vi "Construção string (salvar).vi"(8 "error in (no error)":errorcluster) -> (0 "error out":errorcluster, 2 "String":string)   [LabVIEW 2020]
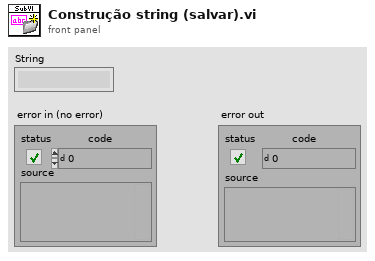
[diagram p1: front panel]
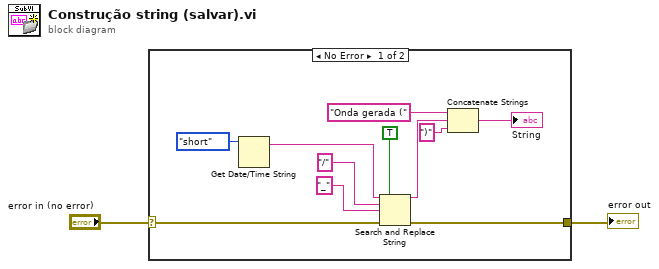
[diagram p0: block diagram]
diagram:
  n1 = case shown="No Error" "error in (no error)" {
    selector: "error in (no error)" -> [w4 w14]
    tunnel: [w3 w14] -> w1
    frame No Error {
      n2 = Get Date/Time String(date format (0)=enum16{"short", "long", "abbreviated"}."short") -> (date string=w12:string)  [unwired: 2 in, 1 out]
      n3 = Search and Replace String(replace all?=TRUE ("replace all? (F)"), input string=w12, search string="/", replace string="_" ("replace string (\"\")"), error in=w4) -> (result string=w13:string, error out=w3:errorcluster)  [unwired: 3 in, 2 out]
      n4 = Concatenate Strings("Onda gerada (" ("string"), w13, ")" ("string")) -> (→"String":string)
    }
    frame Error {
    }
  }
  "error out" <- w1
